vi "Calc - TT1 Avg.vi"(11 "01-01-9213":dbl[](array[numeric])) -> (3 "TT1 Avg":dbl format="%0.2f")   [LabVIEW 2018, in "Controller (Host).lvlib"]
uses:
  Controller (Host).lvlib
  <vilib>/Analysis/baseanly.llb/Mean (DBL).vi
  <vilib>/Analysis/NI_AALBase.lvlib
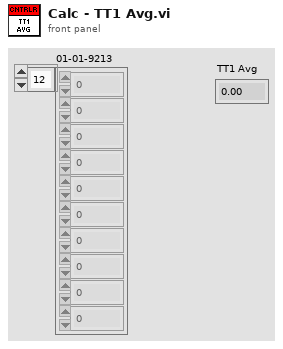
[diagram p1: front panel]
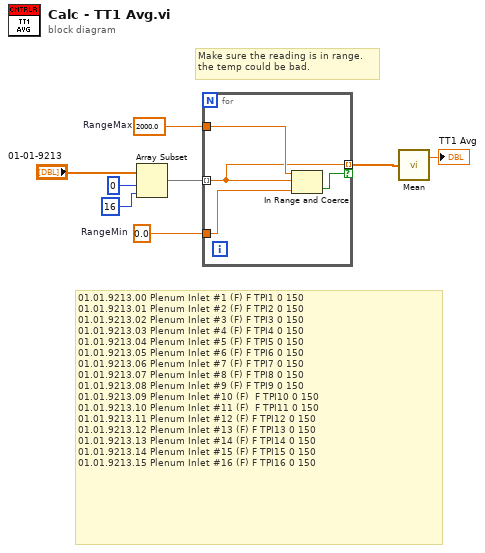
[diagram p0: block diagram]
diagram:
  w3 = 2000.0  # RangeMax
  w4 = 0.0  # RangeMin
  # "01.01.9213.00\tPlenum Inlet #1 (F)\tF\tTPI1\t0\t150\n01.01.9213.01\tPlenum Inlet #2 (F)\tF\tTPI2\t0\t150\n01.01.9213.02\tPlenum Inlet #3 (F)\tF\tTPI3\t0\t150\n01.01.9213.03\tPlenum Inlet #4 (F)\tF\tTPI4\t0\t150\n01.01.9213.04\tPlenum Inlet #5 (F)\tF\tTPI5\t0\t150\n01.01.9213.05\tPlenum Inlet #6 (F)\tF\tTPI6\t0\t150\n01.01.9213.06\tPlenum Inlet #7 (F)\tF\tTPI7\t0\t150\n01.01.9213.07\tPlenum Inlet #8 (F)\tF\tTPI8\t0\t150\n01.01.9213.08\tPlenum Inlet #9 (F)\tF\tTPI9\t0\t150\n01.01.9213.09\tPlenum Inlet #10 (F) \tF\tTPI10\t0\t150\n01.01.9213.10\tPlenum Inlet #11 (F) \tF\tTPI11\t0\t150\n01.01.9213.11\tPlenum Inlet #12 (F)\tF\tTPI12\t0\t150\n01.01.9213.12\tPlenum Inlet #13 (F)\tF\tTPI13\t0\t150\n01.01.9213.13\tPlenum Inlet #14 (F)\tF\tTPI14\t0\t150\n01.01.9213.14\tPlenum Inlet #15 (F)\tF\tTPI15\t0\t150\n01.01.9213.15\tPlenum Inlet #16 (F)\tF\tTPI16\t0\t150"
  # "Make sure the reading is in range. \nthe temp could be bad."
  n1 = Array Subset(array="01-01-9213", index=0, length=16) -> (w5:dbl[])
  n2 = for {
    tunnel: w5 -> [w10] mode=indexing
    tunnel: w4 -> [w11]
    tunnel: w3 -> [w12]
    tunnel: [w10] -> w2 mode=indexing if=w9
    n3 = In Range and Coerce(upper limit=w12, x=w10, lower limit=w11) -> (In Range?=w9:bool)  [unwired: 1 out]
  }
  n4 = call-poly <vilib>:"Mean.vi"("X"=w2) -> ("mean"=→"TT1 Avg":dbl)  [unwired: 1 out]
